vi "Close FrontPanel.vi"(8 "error in (no error)":errorcluster, 11 "VI in":refnum<vi>) -> (0 "error out":errorcluster)   [LabVIEW 2020]
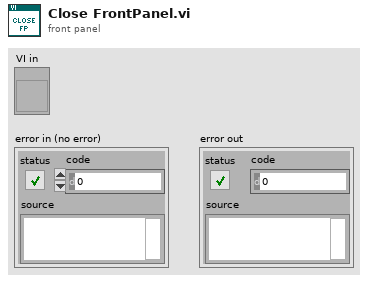
[diagram p1: front panel]
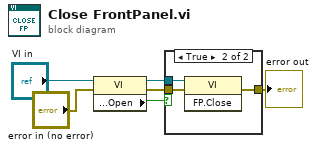
[diagram p0: block diagram]
diagram:
  n1 = property class="VI"(reference="VI in", error in="error in (no error)") -> (reference out=w2:refnum<vi>, error out=w1:errorcluster, "Front Panel.Open"=w3:bool)
  n2 = case shown="True" w3 {
    tunnel: [w7 w10] -> w5
    tunnel: w1 -> [w7 w9]
    tunnel: w2 -> [_ w8]
    frame False {
    }
    frame True {
      n3 = invoke class="VI" method="FP.Close"(reference=w8, error in=w9) -> (error out=w10:errorcluster)  [unwired: 1 in, 2 out]
    }
  }
  "error out" <- w5
